vi "AccessData.vi"(0 "Sensitivity1":i32=1, 4 "CH1Enable":bool, 5 "Sensitivity2":i32=1, 6 "CH2Enable":bool, 7 "Sensitivity3":i32=1, 8 "CH3Enable":bool, 9 "Sensitivity4":i32=1, 10 "CH4Enable":bool, 11 "输入簇":T1, 13 "RmOffset":bool) -> (1 "VibrationWave":dbl[][](array[numeric]) caption="Vibration", 2 "Speed":u16[](array[numeric]), 12 "Error":bool, 15 "输出簇":T1)   [LabVIEW 2012]
uses:
  <vilib>/measure/madcrms.llb/Basic Averaged DC-RMS for 1 Chan.vi
  <vilib>/measure/NI_MAPro.lvlib
panel:
  out "Humidity_Channel":u8
  out "Temperature_Channel7":u8
  out "Temperature_Channel6":dbl
  out "Temperature_Channel5":dbl
  out "Temperature_Channel4":dbl
  out "Temperature_Channel3":dbl
  out "Temperature_Channel2":dbl
  out "Temperature_Channel1":dbl
  out "系统时间":string
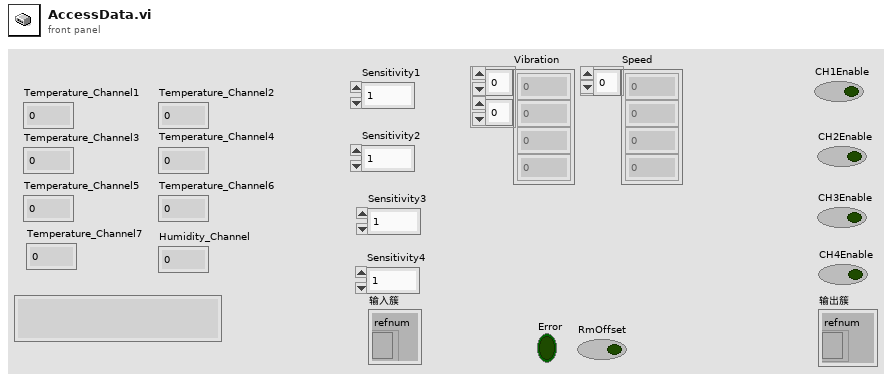
[diagram p1: front panel]
types:
  T1 = cluster{"refnum":refnum<file>, "refnum":refnum<file>, "refnum":refnum<file>, "refnum":refnum<file>, "refnum":refnum<file>, "SavePath":path, "SAVE?":bool, "connection ID":refnum<k5>}
  T2 = enum16{"big-endian, network order", "native, host order", "little-endian"}
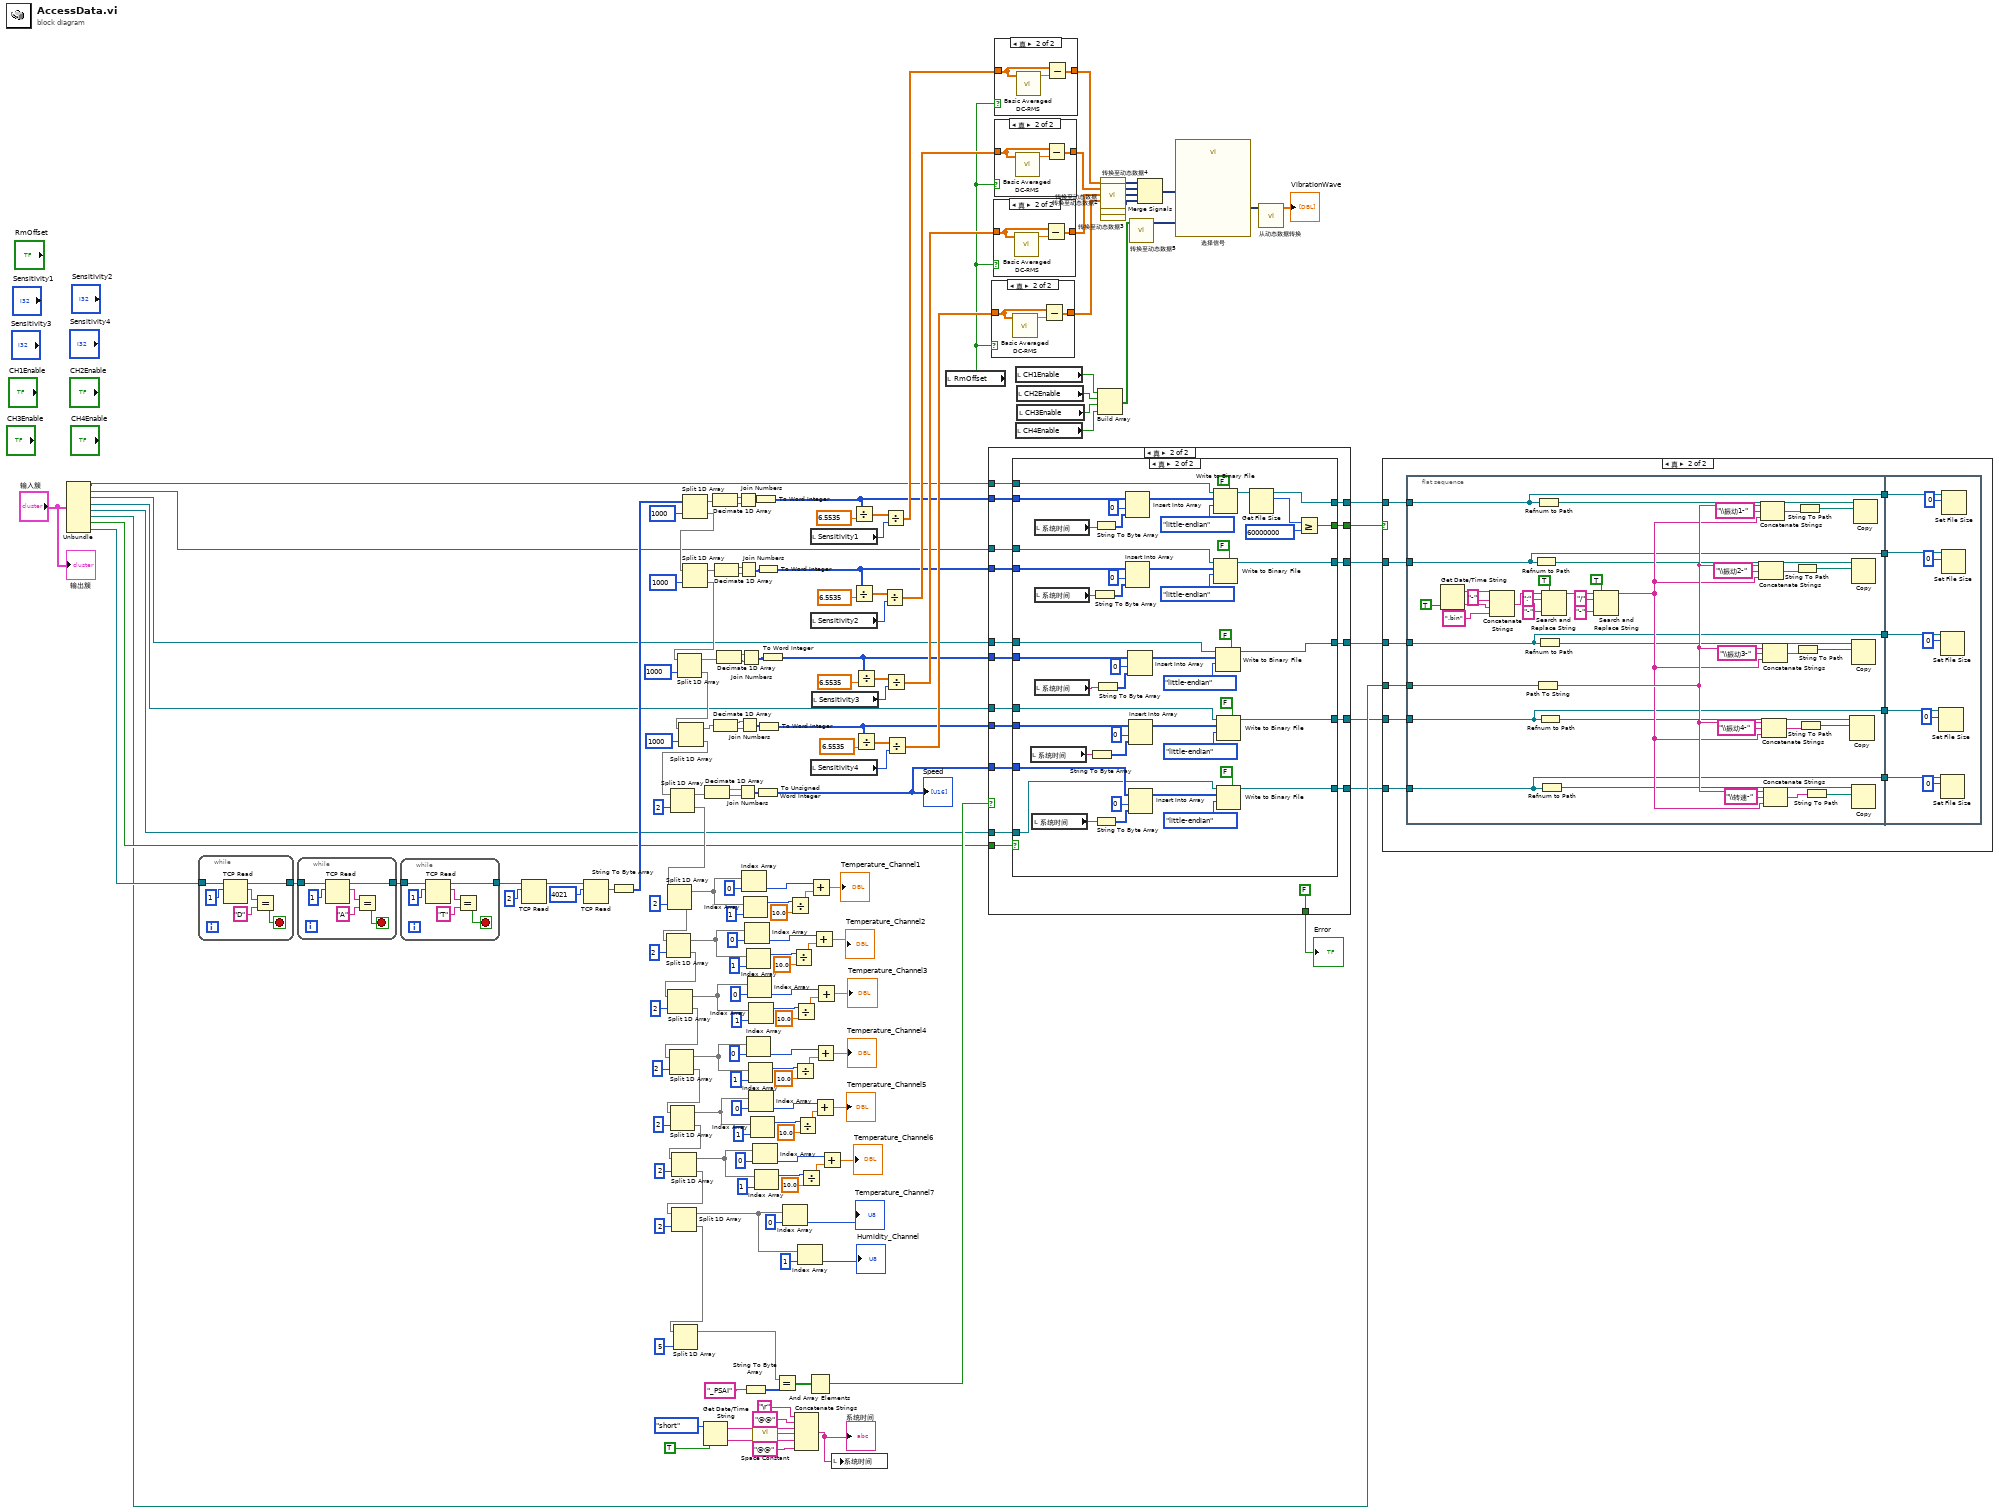
[diagram p0: block diagram]
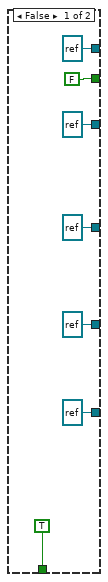
[diagram p6: hidden frame]
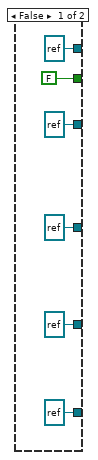
[diagram p7: hidden frame]
diagram:
  n1 = Unbundle("输入簇") -> ("refnum"=w10:refnum<file>, "refnum"=w9:refnum<file>, "refnum"=w8:refnum<file>, "refnum"=w7:refnum<file>, "refnum"=w6:refnum<file>, "SavePath"=w11:path, "SAVE?"=w12:bool, "connection ID"=w13:refnum<k5>)
  n2 = while {
    tunnel: [w178] -> w174
    tunnel: w13 -> [w177]
    stop <- w176 stop-if-true
    n3 = TCP Read(connection ID=w177, bytes to read=1 ("读取的字节")) -> (connection ID out=w178:refnum<k5>, data out=w179:string)  [unwired: 3 in, 1 out]
    n4 = Equal?(x=w179, y="D") -> (x = y?=w176:bool)
  }
  n5 = while {
    tunnel: w174 -> [w187]
    tunnel: [w183] -> w173
    stop <- w182 stop-if-true
    n6 = TCP Read(connection ID=w187, bytes to read=1 ("读取的字节")) -> (connection ID out=w183:refnum<k5>, data out=w186:string)  [unwired: 3 in, 1 out]
    n7 = Equal?(x=w186, y="A") -> (x = y?=w182:bool)
  }
  n8 = while {
    tunnel: w173 -> [w193]
    tunnel: [w189] -> w172
    stop <- w188 stop-if-true
    n9 = TCP Read(connection ID=w193, bytes to read=1 ("读取的字节")) -> (connection ID out=w189:refnum<k5>, data out=w192:string)  [unwired: 3 in, 1 out]
    n10 = Equal?(x=w192, y="T") -> (x = y?=w188:bool)
  }
  n11 = TCP Read(connection ID=w172, bytes to read=2 ("读取的字节")) -> (connection ID out=w45:refnum<k5>)  [unwired: 3 in, 2 out]
  n12 = TCP Read(connection ID=w45, bytes to read=4021 ("最大值(548)")) -> (data out=w156:string)  [unwired: 3 in, 2 out]
  n13 = String To Byte Array(string=w156) -> (unsigned byte array=w155:u8[])
  n14 = Split 1D Array(array=w155, index=1000 ("索引")) -> (first subarray=w85:u8[], second subarray=w82:u8[])
  n15 = Split 1D Array(array=w82, index=1000 ("索引")) -> (first subarray=w81:u8[], second subarray=w78:u8[])
  n16 = Split 1D Array(array=w78, index=1000 ("索引")) -> (first subarray=w77:u8[], second subarray=w76:u8[])
  n17 = Split 1D Array(array=w76, index=1000 ("索引")) -> (first subarray=w73:u8[], second subarray=w86:u8[])
  n18 = Split 1D Array(array=w86, index=2 ("索引")) -> (first subarray=w70:u8[], second subarray=w145:u8[])
  n19 = Split 1D Array(array=w145, index=2 ("索引")) -> (first subarray=w128:u8[], second subarray=w144:u8[])
  n20 = Split 1D Array(array=w144, index=2 ("索引")) -> (first subarray=w92:u8[], second subarray=w143:u8[])
  n21 = Split 1D Array(array=w143, index=2 ("索引")) -> (first subarray=w91:u8[], second subarray=w130:u8[])
  n22 = Split 1D Array(array=w130, index=2 ("索引")) -> (first subarray=w90:u8[], second subarray=w139:u8[])
  n23 = Split 1D Array(array=w139, index=2 ("索引")) -> (first subarray=w89:u8[], second subarray=w138:u8[])
  n24 = Split 1D Array(array=w138, index=2 ("索引")) -> (first subarray=w88:u8[], second subarray=w129:u8[])
  n25 = Split 1D Array(array=w129, index=2 ("索引")) -> (first subarray=w87:u8[], second subarray=w65:u8[])
  n26 = Split 1D Array(array=w65, index=5 ("索引")) -> (first subarray=w64:u8[])  [unwired: 1 out]
  n27 = Get Date/Time String(date format (0)=enum16{"short", "long", "abbreviated"}."short" ("日期格式(0)"), want seconds? (F)=TRUE ("需要秒？(F)")) -> (date string=w152:string, time string=w146:string)  [unwired: 1 in]
  n28 = Decimate 1D Array(w70) -> (w69:u8[], w68:u8[])
  n29 = Decimate 1D Array(w85) -> (w84:u8[], w83:u8[])
  n30 = Decimate 1D Array(w73) -> (w72:u8[], w71:u8[])
  n31 = Decimate 1D Array(w81) -> (w80:u8[], w79:u8[])
  n32 = Decimate 1D Array(w77) -> (w75:u8[], w74:u8[])
  n33 = Join Numbers(hi=w69, lo=w68) -> ((hi.lo)=w67:u16[])
  n34 = Join Numbers(hi=w84, lo=w83) -> ((hi.lo)=w168:u16[])
  n35 = Join Numbers(hi=w80, lo=w79) -> ((hi.lo)=w163:u16[])
  n36 = Join Numbers(hi=w72, lo=w71) -> ((hi.lo)=w165:u16[])
  n37 = Join Numbers(hi=w75, lo=w74) -> ((hi.lo)=w164:u16[])
  n38 = Index Array(array=w128, index=0 ("索引")) -> (element=w123:u8)
  n39 = Index Array(array=w128, index=1 ("索引")) -> (element=w125:u8)
  n40 = String To Byte Array(string="_PSAI") -> (unsigned byte array=w159:u8[])
  n41 = Index Array(array=w92, index=0 ("索引")) -> (element=w117:u8)
  n42 = Index Array(array=w92, index=1 ("索引")) -> (element=w119:u8)
  n43 = Index Array(array=w90, index=0 ("索引")) -> (element=w105:u8)
  n44 = Index Array(array=w91, index=0 ("索引")) -> (element=w111:u8)
  n45 = Index Array(array=w90, index=1 ("索引")) -> (element=w107:u8)
  n46 = Index Array(array=w91, index=1 ("索引")) -> (element=w113:u8)
  n47 = Index Array(array=w89, index=0 ("索引")) -> (element=w99:u8)
  n48 = Index Array(array=w89, index=1 ("索引")) -> (element=w101:u8)
  n49 = Index Array(array=w88, index=0 ("索引")) -> (element=w93:u8)
  n50 = call <vilib>:"Space Constant.vi"() -> ("String"=w148:string)
  n51 = To Word Integer(number=w168) -> (16bit integer=w18:i16[])
  n52 = Index Array(array=w88, index=1 ("索引")) -> (element=w95:u8)
  n53 = To Unsigned Word Integer(number=w67) -> (unsigned 16bit integer=w63:u16[])
  "Speed" <- w63
  n54 = To Word Integer(number=w163) -> (16bit integer=w17:i16[])
  n55 = To Word Integer(number=w165) -> (16bit integer=w15:i16[])
  n56 = To Word Integer(number=w164) -> (16bit integer=w16:i16[])
  n57 = Equal?(x=w64, y=w159) -> (x = y?=w158:bool[])
  n58 = Index Array(array=w87, index=0 ("索引")) -> (element=→"Temperature_Channel7":u8)
  n59 = Divide(x=w125, y=10.0) -> (x/y=w124:dbl)
  n60 = Divide(x=w119, y=10.0) -> (x/y=w118:dbl)
  n61 = Divide(x=w107, y=10.0) -> (x/y=w106:dbl)
  n62 = Divide(x=w113, y=10.0) -> (x/y=w112:dbl)
  n63 = Concatenate Strings("\r", "@@" ("字符串"), w152, w148, w146, "@@" ("字符串")) -> (w151:string)
  "系统时间" <- w151
  n64 = Divide(x=w101, y=10.0) -> (x/y=w100:dbl)
  n65 = Index Array(array=w87, index=1 ("索引")) -> (element=→"Humidity_Channel":u8)
  n66 = Divide(x=w95, y=10.0) -> (x/y=w94:dbl)
  n67 = And Array Elements(Boolean array=w158) -> (logical AND=w157:bool)
  n68 = Add(x=w123, y=w124) -> (x+y=→"Temperature_Channel1":dbl)
  n69 = local read "Sensitivity1"() -> (w44:i32)
  n70 = local read "Sensitivity2"() -> (w43:i32)
  n71 = local read "Sensitivity4"() -> (w41:i32)
  n72 = local read "Sensitivity3"() -> (w42:i32)
  n73 = Add(x=w117, y=w118) -> (x+y=→"Temperature_Channel2":dbl)
  n74 = Add(x=w99, y=w100) -> (x+y=→"Temperature_Channel5":dbl)
  n75 = Add(x=w105, y=w106) -> (x+y=→"Temperature_Channel4":dbl)
  n76 = Add(x=w111, y=w112) -> (x+y=→"Temperature_Channel3":dbl)
  n77 = Add(x=w93, y=w94) -> (x+y=→"Temperature_Channel6":dbl)
  n78 = local write "系统时间"(w151) -> ()
  n79 = Divide(x=w18, y=6.5535) -> (x/y=w55:dbl[])
  n80 = Divide(x=w17, y=6.5535) -> (x/y=w56:dbl[])
  n81 = Divide(x=w16, y=6.5535) -> (x/y=w57:dbl[])
  n82 = Divide(x=w15, y=6.5535) -> (x/y=w58:dbl[])
  n83 = Divide(x=w56, y=w43) -> (x/y=w40:dbl[])
  n84 = Divide(x=w55, y=w44) -> (x/y=w23:dbl[])
  n85 = Divide(x=w57, y=w42) -> (x/y=w39:dbl[])
  n86 = Divide(x=w58, y=w41) -> (x/y=w38:dbl[])
  n87 = local read "RmOffset"() -> (w37:bool)
  n88 = case shown="真" w157 {
    tunnel: [TRUE FALSE] -> w46
    tunnel: w18 -> [_ w218]
    tunnel: w17 -> [_ w217]
    tunnel: w16 -> [_ w216]
    tunnel: w15 -> [_ w215]
    tunnel: w63 -> [_ w214]
    tunnel: w10 -> [_ w212]
    tunnel: w9 -> [_ w211]
    tunnel: w8 -> [_ w210]
    tunnel: w7 -> [_ w209]
    tunnel: w6 -> [_ w208]
    tunnel: w12 -> [_ w207]
    tunnel: [FALSE w206] -> w175
    tunnel: [refnum<file> refnum ("refnum out") w205] -> w5
    tunnel: [refnum<file> refnum ("refnum out") w204] -> w4
    tunnel: [refnum<file> refnum ("refnum out") w203] -> w3
    tunnel: [refnum<file> refnum ("refnum out") w202] -> w2
    tunnel: [refnum<file> refnum ("refnum out") w201] -> w1
    frame False {
    }
    frame True {
      n89 = case shown="真" w207 {
        tunnel: w218 -> [_ w272]
        tunnel: w217 -> [_ w252]
        tunnel: w216 -> [_ w251]
        tunnel: w215 -> [_ w250]
        tunnel: w214 -> [_ w249]
        tunnel: w212 -> [_ w238]
        tunnel: w211 -> [_ w237]
        tunnel: w210 -> [_ w236]
        tunnel: w209 -> [_ w235]
        tunnel: w208 -> [_ w234]
        tunnel: [FALSE w231] -> w206
        tunnel: [refnum<file> refnum ("refnum out") w229] -> w205
        tunnel: [refnum<file> refnum ("refnum out") w228] -> w204
        tunnel: [refnum<file> refnum ("refnum out") w227] -> w203
        tunnel: [refnum<file> refnum ("refnum out") w226] -> w202
        tunnel: [refnum<file> refnum ("refnum out") w225] -> w201
        frame False {
        }
        frame True {
          n90 = local read "系统时间"() -> (w246:string)
          n91 = local read "系统时间"() -> (w248:string)
          n92 = local read "系统时间"() -> (w240:string)
          n93 = local read "系统时间"() -> (w242:string)
          n94 = local read "系统时间"() -> (w244:string)
          n95 = String To Byte Array(string=w246) -> (unsigned byte array=w245:u8[])
          n96 = String To Byte Array(string=w242) -> (unsigned byte array=w241:u8[])
          n97 = String To Byte Array(string=w240) -> (unsigned byte array=w239:u8[])
          n98 = String To Byte Array(string=w248) -> (unsigned byte array=w247:u8[])
          n99 = String To Byte Array(string=w244) -> (unsigned byte array=w243:u8[])
          n100 = Insert Into Array(array=w272, index=0 ("索引"), new element=w239) -> (w270:i16[])
          n101 = Insert Into Array(array=w252, index=0 ("索引"), new element=w241) -> (w266:i16[])
          n102 = Insert Into Array(array=w251, index=0 ("索引"), new element=w243) -> (w262:i16[])
          n103 = Insert Into Array(array=w250, index=0 ("索引"), new element=w245) -> (w258:i16[])
          n104 = Insert Into Array(array=w249, index=0 ("索引"), new element=w247) -> (w254:u16[])
          n105 = Write to Binary File(file (use dialog)=w238, data=w270, 5:FALSE ("预置数组或字符串大小？(T)"), 9:T2."little-endian" ("字节顺序(0:big-endian, network order)")) -> (refnum out=w230:refnum<file>)  [unwired: 2 in, 2 out]
          n106 = Write to Binary File(file (use dialog)=w237, data=w266, 5:FALSE ("预置数组或字符串大小？(T)"), 9:T2."little-endian" ("字节顺序(0:big-endian, network order)")) -> (refnum out=w228:refnum<file>)  [unwired: 2 in, 2 out]
          n107 = Write to Binary File(file (use dialog)=w236, data=w262, 5:FALSE ("预置数组或字符串大小？(T)"), 9:T2."little-endian" ("字节顺序(0:big-endian, network order)")) -> (refnum out=w227:refnum<file>)  [unwired: 2 in, 2 out]
          n108 = Write to Binary File(file (use dialog)=w235, data=w258, 5:FALSE ("预置数组或字符串大小？(T)"), 9:T2."little-endian" ("字节顺序(0:big-endian, network order)")) -> (refnum out=w226:refnum<file>)  [unwired: 2 in, 2 out]
          n109 = Write to Binary File(file (use dialog)=w234, data=w254, 5:FALSE ("预置数组或字符串大小？(T)"), 9:T2."little-endian" ("字节顺序(0:big-endian, network order)")) -> (refnum out=w225:refnum<file>)  [unwired: 2 in, 2 out]
          n110 = Get File Size(file=w230) -> (refnum out=w229:refnum<file>, size (in bytes)=w233:i64)  [unwired: 1 in, 1 out]
          n111 = Greater Or Equal?(x=w233, y=i64 60000000) -> (x >= y?=w231:bool)
        }
      }
    }
  }
  "Error" <- w46
  n112 = case shown="真" w37 {
    tunnel: w38 -> [w274 w275]
    tunnel: [w274 w276] -> w26
    frame False {
    }
    frame True {
      n113 = call-poly <vilib>:"Basic Averaged DC-RMS.vi"("signal in"=w275) -> ("DC value"=w277:dbl)  [unwired: 7 in, 3 out]
      n114 = Subtract(x=w275, y=w277) -> (x-y=w276:dbl[])
    }
  }
  n115 = case shown="真" w37 {
    tunnel: w39 -> [w278 w279]
    tunnel: [w278 w280] -> w28
    frame False {
    }
    frame True {
      n116 = call-poly <vilib>:"Basic Averaged DC-RMS.vi"("signal in"=w279) -> ("DC value"=w281:dbl)  [unwired: 7 in, 3 out]
      n117 = Subtract(x=w279, y=w281) -> (x-y=w280:dbl[])
    }
  }
  n118 = case shown="真" w37 {
    tunnel: w40 -> [w282 w283]
    tunnel: [w282 w284] -> w30
    frame False {
    }
    frame True {
      n119 = call-poly <vilib>:"Basic Averaged DC-RMS.vi"("signal in"=w283) -> ("DC value"=w285:dbl)  [unwired: 7 in, 3 out]
      n120 = Subtract(x=w283, y=w285) -> (x-y=w284:dbl[])
    }
  }
  n121 = case shown="真" w37 {
    tunnel: w23 -> [w286 w287]
    tunnel: [w286 w288] -> w22
    frame False {
    }
    frame True {
      n122 = call-poly <vilib>:"Basic Averaged DC-RMS.vi"("signal in"=w287) -> ("DC value"=w289:dbl)  [unwired: 7 in, 3 out]
      n123 = Subtract(x=w287, y=w289) -> (x-y=w288:dbl[])
    }
  }
  n124 = local read "CH1Enable"() -> (w32:bool)
  n125 = local read "CH4Enable"() -> (w33:bool)
  n126 = local read "CH2Enable"() -> (w35:bool)
  n127 = local read "CH3Enable"() -> (w34:bool)
  n128 = Build Array(w32, w35, w34, w33) -> (w31:bool[])
  n129 = call "转换至动态数据4"("Array"=w22) -> ("Dynamic Data Type"=w24:dynamicdata)  [unwired: 3 in]
  n130 = call "转换至动态数据"("Array"=w30) -> ("Dynamic Data Type"=w29:dynamicdata)  [unwired: 3 in]
  n131 = call "转换至动态数据2"("Array"=w28) -> ("Dynamic Data Type"=w27:dynamicdata)  [unwired: 3 in]
  n132 = call "转换至动态数据3"("Array"=w26) -> ("Dynamic Data Type"=w25:dynamicdata)  [unwired: 3 in]
  n133 = call "转换至动态数据5"("Array"=w31) -> ("Dynamic Data Type"=w36:dynamicdata)  [unwired: 3 in]
  n134 = Merge Signals(w24, w29, w27, w25) -> (w21:dynamicdata)
  n135 = call "选择信号"("Selector Input"=w36, "Signals"=w21) -> ("Signal Out"=w20:dynamicdata)  [unwired: 8 in, 1 out]
  n136 = call "从动态数据转换"("Dynamic Data Type"=w20) -> ("Array"=→"VibrationWave":dbl[][])  [unwired: 3 in]
  n137 = case shown="真" w175 {
    tunnel: w11 -> [_ w300]
    tunnel: w5 -> [_ w299]
    tunnel: w4 -> [_ w298]
    tunnel: w3 -> [_ w297]
    tunnel: w2 -> [_ w296]
    tunnel: w1 -> [_ w295]
    frame False {
    }
    frame True {
      n138 = flat-sequence {
        tunnel: w300 -> [w310]
        tunnel: w299 -> [w305]
        tunnel: w298 -> [w304]
        tunnel: w297 -> [w303]
        tunnel: w296 -> [w302]
        tunnel: w295 -> [w301]
        tunnel: [w305] -> w294
        tunnel: [w304] -> w293
        tunnel: [w303] -> w292
        tunnel: [w302] -> w291
        tunnel: [w301] -> w290
        tunnel: w294 -> [w346]
        tunnel: w293 -> [w345]
        tunnel: w292 -> [w344]
        tunnel: w291 -> [w343]
        tunnel: w290 -> [w342]
        frame #0 {
          n139 = Get Date/Time String(want seconds? (F)=TRUE ("需要秒？(F)")) -> (date string=w329:string, time string=w326:string)  [unwired: 2 in]
          n140 = Concatenate Strings(w329, "-" ("字符串"), w326, ".bin" ("字符串")) -> (w325:string)
          n141 = Refnum to Path(1:w304) -> (0:w309:path)
          n142 = Path To String(path=w310) -> (string=w336:string)
          n143 = Refnum to Path(1:w305) -> (0:w316:path)
          n144 = Refnum to Path(1:w303) -> (0:w308:path)
          n145 = Refnum to Path(1:w302) -> (0:w307:path)
          n146 = Refnum to Path(1:w301) -> (0:w306:path)
          n147 = Search and Replace String(replace all?=TRUE ("替换全部？(F)"), input string=w325, search string=":" ("搜索字符串"), replace string="-" ("替换字符串(\"\")")) -> (result string=w318:string)  [unwired: 4 in, 3 out]
          n148 = Search and Replace String(replace all?=TRUE ("替换全部？(F)"), input string=w318, search string="/" ("搜索字符串"), replace string="-" ("替换字符串(\"\")")) -> (result string=w317:string)  [unwired: 4 in, 3 out]
          n149 = Concatenate Strings(w336, "\\振动2-" ("字符串"), w317) -> (w338:string)
          n150 = Concatenate Strings(w336, "\\振动1-" ("字符串"), w317) -> (w337:string)
          n151 = Concatenate Strings(w336, "\\振动4-" ("字符串"), w317) -> (w340:string)
          n152 = Concatenate Strings(w336, "\\振动3-" ("字符串"), w317) -> (w339:string)
          n153 = Concatenate Strings(w336, "\\转速-" ("字符串"), w317) -> (w341:string)
          n154 = String To Path(string=w338) -> (path=w314:path)
          n155 = String To Path(string=w339) -> (path=w313:path)
          n156 = String To Path(string=w337) -> (path=w315:path)
          n157 = String To Path(string=w340) -> (path=w312:path)
          n158 = String To Path(string=w341) -> (path=w311:path)
          n159 = Copy(10:w312, 11:w307) -> ()  [unwired: 3 in, 3 out]
          n160 = Copy(10:w314, 11:w309) -> ()  [unwired: 3 in, 3 out]
          n161 = Copy(10:w313, 11:w308) -> ()  [unwired: 3 in, 3 out]
          n162 = Copy(10:w311, 11:w306) -> ()  [unwired: 3 in, 3 out]
          n163 = Copy(10:w315, 11:w316) -> ()  [unwired: 3 in, 3 out]
        }
        frame #1 {
          n164 = Set File Size(6:i64 0 ("大小（字节）"), 7:w343) -> ()  [unwired: 1 in, 2 out]
          n165 = Set File Size(6:i64 0 ("大小（字节）"), 7:w344) -> ()  [unwired: 1 in, 2 out]
          n166 = Set File Size(6:i64 0 ("大小（字节）"), 7:w342) -> ()  [unwired: 1 in, 2 out]
          n167 = Set File Size(6:i64 0 ("大小（字节）"), 7:w345) -> ()  [unwired: 1 in, 2 out]
          n168 = Set File Size(6:i64 0 ("大小（字节）"), 7:w346) -> ()  [unwired: 1 in, 2 out]
        }
      }
    }
  }
  "输出簇" <- "输入簇"
